vi "Add Data Replay.vi"(4 "DataReplay":T2, 8 "error in (no error)":errorcluster, 11 "Section Ptr":T1 format="%.0x") -> (0 "error out":errorcluster)   [LabVIEW 2011, in "Engine Sim System Explorer.lvlib"]
uses:
  Engine Sim System Explorer.lvlib
  TypeDefs/DataReplayComp.ctl
  <vilib>/NI Veristand/Custom Device API/Custom Device Item Ref.ctl
  <vilib>/NI Veristand/Custom Device API/Custom Device Channel.ctl
  <vilib>/NI Veristand/Custom Device API/Custom Device Channel Type.ctl
  Shared/Engine Simulation Global.vi
  <vilib>/NI Veristand/Custom Device API/Set Item Property (Boolean).vi
  <vilib>/NI Veristand/Custom Device API/Custom Device API.lvlib
  Engine Simulation Shared.lvlib
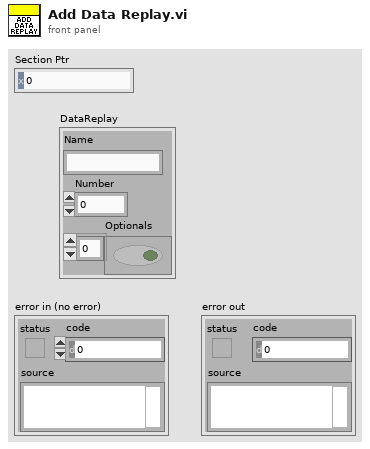
[diagram p1: front panel]
types:
  T1 = typedef "Custom Device API.lvlib/Custom Device Item Ref.ctl" = u64
  T2 = typedef "Engine Sim System Explorer.lvlib/DataReplayComp.ctl" = cluster{"Name":string, "Number":i32, "Optionals":bool[]}
  T3 = typedef "Custom Device API.lvlib/Custom Device Channel.ctl" = cluster{"Type":T4, "Units":string, "Default Value":dbl, "Faultable":bool, "Scalable":bool}
  T4 = typedef "Custom Device API.lvlib/Custom Device Channel Type.ctl" = enum16{"Input", "Output"}
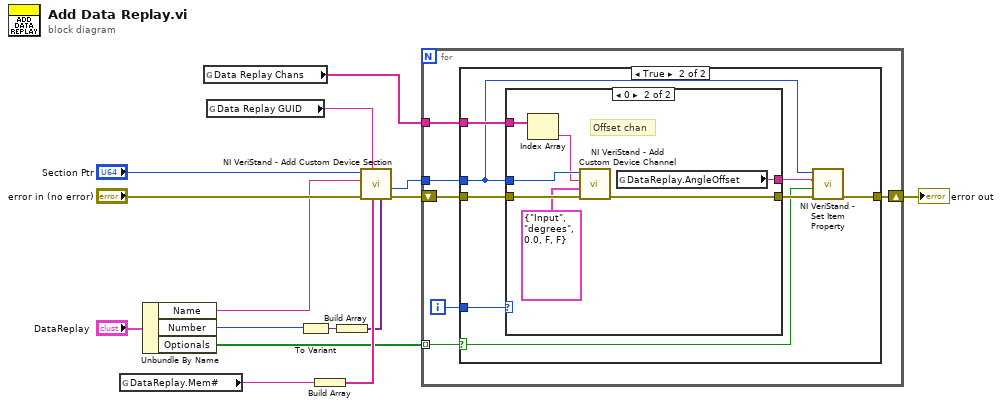
[diagram p0: block diagram]
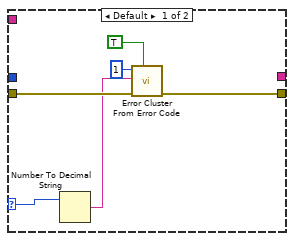
[diagram p3: hidden frame]
diagram:
  n1 = global read "Engine Simulation Global.vi" "DataReplay.Mem#"() -> (w12:string)
  n2 = Unbundle By Name("DataReplay") -> ("Name"=w9:string, "Number"=w7:i32, "Optionals"=w1:bool[])
  n3 = global read "Engine Simulation Global.vi" "Data Replay Chans"() -> (w2:string[])
  n4 = global read "Engine Simulation Global.vi" "Data Replay GUID"() -> (w11:string)
  n5 = To Variant(anything=w7) -> (Variant=w8:variant)
  n6 = Build Array(w12) -> (w10:string[])
  n7 = Build Array(w8) -> (w6:variant[])
  n8 = call <vilib>:"NI VeriStand - Add Custom Device Section.vi"("Property Values"=w6, "Property names"=w10, "GUID (Default Section)"=w11, "error in (no error)"="error in (no error)", "Section Name"=w9, "Parent Ref in"="Section Ptr") -> ("error out"=w5:errorcluster, "Section Ptr"=w4:T1)  [unwired: 2 in, 2 out]
  n9 = for {
    shift-right: [w19] -> w3
    shift-left: w5 -> [w21]
    tunnel: w1 -> [w18] mode=indexing
    tunnel: w4 -> [w20]
    tunnel: w2 -> [w16]
    i -> [w17]
    n10 = case shown="True" w18 {
      selector: w18 -> [_ w24]
      tunnel: w21 -> [w22 w30]
      tunnel: w20 -> [_ w23]
      tunnel: [w22 w26] -> w19
      tunnel: w17 -> [_ w28]
      tunnel: w16 -> [_ w27]
      frame False {
      }
      frame True {
        n11 = case shown="0" w28 {
          selector: w28 -> [w32 _]
          tunnel: w30 -> [w36 w43]
          tunnel: w23 -> [_ w42]
          tunnel: [w35 w41] -> w29
          tunnel: w27 -> [_ w40]
          tunnel: [_ w38] -> w25
          frame Default {
            n12 = Number To Decimal String(number=w32) -> (decimal integer string=w31:string)  [unwired: 1 in]
            n13 = call <vilib>:"Error Cluster From Error Code.vi"("show call chain? (False)"=TRUE, "error in (no error)"=w36, "error message (\"\")"=w31, "error code (0)"=1) -> ("error out"=w35:errorcluster)  [unwired: 5 in]
          }
          frame 0 {
            # "Offset chan"
            n14 = Index Array(array=w40) -> (element=w39:string)  [unwired: 1 in]
            n15 = call <vilib>:"NI VeriStand - Add Custom Device Channel.vi"("error in (no error)"=w43, "Channel"=T3 {"Type"=enum."Input", "Units"="degrees", "Default Value"=0.0, "Faultable"=FALSE, "Scalable"=FALSE}, "Channel Name"=w39, "Parent Ref in"=w42) -> ("error out"=w41:errorcluster)  [unwired: 4 in, 3 out]
            n16 = global read "Engine Simulation Global.vi" "DataReplay.AngleOffset"() -> (w38:string)
          }
        }
        n17 = call-poly <vilib>:"NI VeriStand - Set Item Property.vi"("error in (no error)"=w29, "Value"=w24, "Property Name"=w25, "Item Ref in"=w23) -> ("error out"=w26:errorcluster)  [unwired: 5 in, 2 out]
      }
    }
  }
  "error out" <- w3
